vi "Fixed Heading.vi"(2 "inputRotation":dbl, 3 "joystickHeading(x,y)":cluster{"X":dbl, "Y":dbl}) -> (0 "outputRotation":dbl)   [LabVIEW 2019]
uses:
  swerveData.vi
  <vilib>/addons/control/pid/pid.llb/PID (DBL).vi
  <vilib>/addons/control/pid/NI_PID_pid.lvlib
panel:
  in  "headingStay":dbl
  in  "heading":T1={"proportional gain (Kc)"=10.0, "integral time (Ti, min)"=0.0, "derivative time (Td, min)"=0.7} {"derivative time (Td, min)" format="%.3f"; "integral time (Ti, min)" format="%.3f"; "proportional gain (Kc)" format="%.3f"}
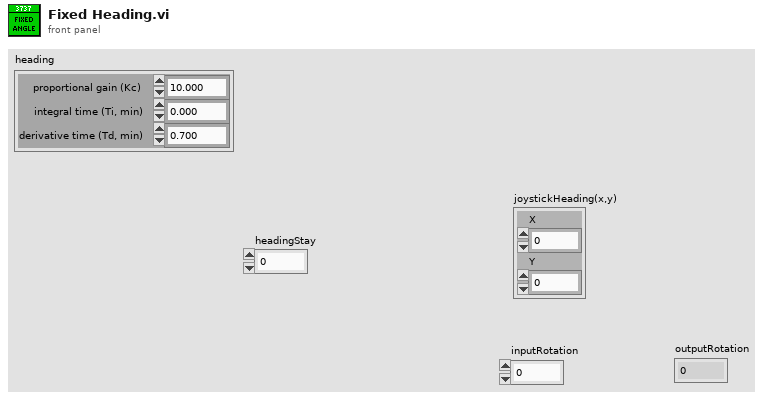
[diagram p1: front panel]
types:
  T1 = cluster{"proportional gain (Kc)":dbl, "integral time (Ti, min)":dbl, "derivative time (Td, min)":dbl}
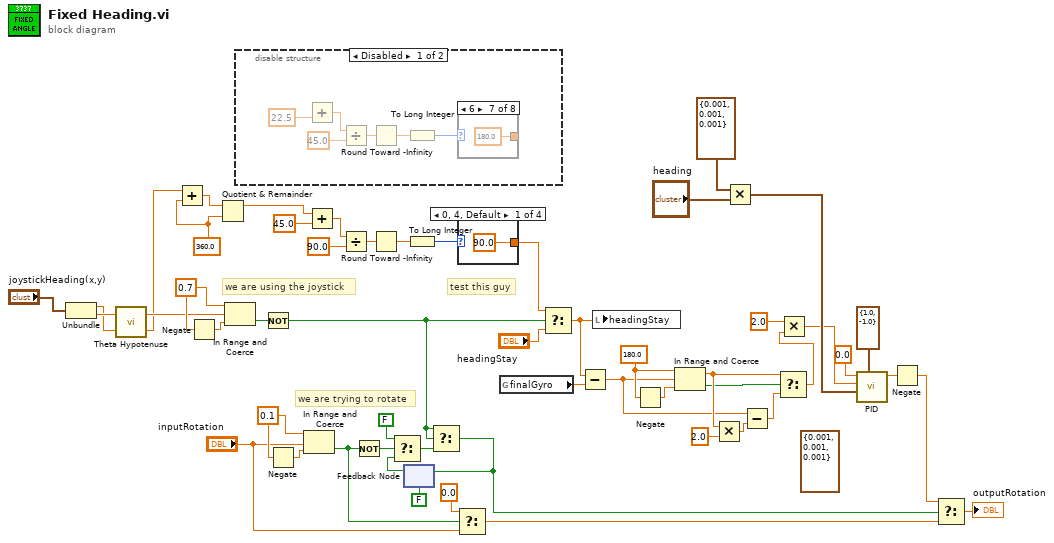
[diagram p0: block diagram]
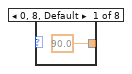
[diagram p2: hidden frame]
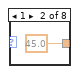
[diagram p3: hidden frame]
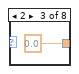
[diagram p4: hidden frame]
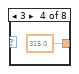
[diagram p5: hidden frame]
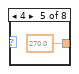
[diagram p6: hidden frame]
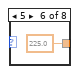
[diagram p7: hidden frame]
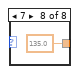
[diagram p8: hidden frame]
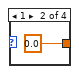
[diagram p10: hidden frame]
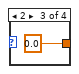
[diagram p11: hidden frame]
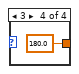
[diagram p12: hidden frame]
diagram:
  (unwired) T1 {"proportional gain (Kc)"=0.001, "integral time (Ti, min)"=0.001, "derivative time (Td, min)"=0.001} ("x")
  w25 = 180.0
  w33 = 0.7 ("lower limit")
  w38 = 360.0 ("y")
  w53 = 0.1 ("lower limit")
  # "test this guy"
  # "we are trying to rotate"
  # "we are using the joystick"
  n1 = Unbundle("joystickHeading(x,y)") -> ("X"=w28:dbl, "Y"=w29:dbl)
  n2 = call "Theta Hypotenuse.vi"("x value"=w28, "y value"=w29) -> ("Theta"=w30:dbl, "Hypotenuse"=w31:dbl)
  n3 = Add(x=w30, y=w38) -> (x+y=w39:dbl)
  n4 = Negate(x=w33) -> (-x=w34:dbl)
  n5 = Quotient & Remainder(x=w39, y=w38) -> (x-y*floor(x/y)=w35:dbl)  [unwired: 1 out]
  n6 = In Range and Coerce(upper limit=w33, x=w31, lower limit=w34) -> (In Range?=w32:bool)  [unwired: 1 out]
  n7 = disable-structure shown="Disabled" {
    frame Disabled {
      n8 = Add(y=22.5) -> (x+y=w56:dbl)  [unwired: 1 in]
      n9 = Divide(x=w56, y=45.0) -> (x/y=w57:dbl)
      n10 = Round Toward -Infinity(1:w57) -> (0:w58:dbl)
      n11 = To Long Integer(number=w58) -> (32bit integer=w59:i32)
      n12 = case shown="6" w59 {
        tunnel: [90.0 45.0 0.0 315.0 270.0 225.0 180.0 135.0] -> _
        frame 0, 8, Default {
        }
        frame 1 {
        }
        frame 2 {
        }
        frame 3 {
        }
        frame 4 {
        }
        frame 5 {
        }
        frame 6 {
        }
        frame 7 {
        }
      }
    }
    frame Enabled {
    }
  }
  n13 = Not(x=w32) -> (.not. x?=w14:bool)
  n14 = Negate(x=w53) -> (-x=w52:dbl)
  n15 = In Range and Coerce(upper limit=w53, x="inputRotation", lower limit=w52) -> (In Range?=w7:bool)  [unwired: 1 out]
  n16 = Add(x=w35, y=45.0) -> (x+y=w45:dbl)
  n17 = Divide(x=w45, y=90.0) -> (x/y=w44:dbl)
  n18 = Not(x=w7) -> (.not. x?=w13:bool)
  n19 = Round Toward -Infinity(1:w44) -> (0:w43:dbl)
  n20 = feedback #1(FALSE) -> (w10:bool)
  n21 = Select(t=FALSE, s=w13, f=w10) -> (s? t:f=w11:bool)
  n22 = To Long Integer(number=w43) -> (32bit integer=w26:i32)
  n23 = Select(t=w14, s=w14, f=w11) -> (s? t:f=w8:bool)
  n24 = feedback-in #1(w8) -> ()
  n25 = Select(t=0.0, s=w7, f="inputRotation") -> (s? t:f=w4:dbl)
  n26 = case shown="0, 4, Default" w26 {
    tunnel: [90.0 0.0 0.0 180.0] -> w42
    frame 0, 4, Default {
    }
    frame 1 {
    }
    frame 2 {
    }
    frame 3 {
    }
  }
  n27 = global read "swerveData.vi" "finalGyro"() -> (w27:dbl)
  n28 = Select(t=w42, s=w14, f="headingStay") -> (s? t:f=w37:dbl)
  n29 = Subtract(x=w37, y=w27) -> (x-y=w19:dbl)
  n30 = local write "headingStay"(w37) -> ()
  n31 = Negate(x=w25) -> (-x=w24:dbl)
  n32 = In Range and Coerce(upper limit=w25, x=w19, lower limit=w24) -> (coerced(x)=w21:dbl, In Range?=w18:bool)
  n33 = Multiply(x=w21, y=2.0) -> (x*y=w22:dbl)
  n34 = Multiply(x=T1 {"proportional gain (Kc)"=0.001, "integral time (Ti, min)"=0.001, "derivative time (Td, min)"=0.001}, y="heading") -> (x*y=w50:T1)
  n35 = Subtract(x=w19, y=w22) -> (x-y=w23:dbl)
  n36 = Select(t=w21, s=w18, f=w23) -> (s? t:f=w3:dbl)
  n37 = Multiply(x=2.0, y=w3) -> (x*y=w1:dbl)
  n38 = call-poly <vilib>:"PID.vi"("output range"=cluster{"output high":dbl, "output low":dbl} {"output high"=1.0, "output low"=-1.0}, "PID gains"=w50, "process variable"=w1, "setpoint"=0.0) -> ("output"=w16:dbl)  [unwired: 6 in, 1 out]
  n39 = Negate(x=w16) -> (-x=w17:dbl)
  n40 = Select(t=w17, s=w8, f=w4) -> (s? t:f=→"outputRotation":dbl)
